vi "Blood Flow Measurement.vi"() -> ()   [LabVIEW 2023]
doc: "This example shows the application of the Time Frequency Analysis VIs in blood flow measurement. \n\nBlood velocity within a vessel is not uniform. Blood flow often has the maximum velocity at the center of a vessel and a zero velocity at the vascular wall. Blood velocity also changes over time. The complexity of the velocity distribution in a vessel is often associated with some arterial diseases. For example, when there is a high-grade stenosis within a femoral artery, the blood flow at the outlet of the stenosis usually has a velocity of a large mean, while the vortex or turbulence at the downstream generates a complicated velocity distribution. \n\nThe Doppler ultrasound technique has been widely applied to non-invasive blood flow measurement. The Doppler signals are generated by the backscattering from moving blood cells. The mean instantaneous frequency of the detected Doppler signal is proportional to the mean blood flow velocity in a vessel. The mean instantaneous bandwidth of the Doppler signal describes the velocity variation of the blood flow. \n\nThis example computes the time-frequency representation of a simulated Doppler signal and estimates the velocity and frequency bandwidth of the signal using the mean instantaneous frequency and mean instantaneous bandwidth of the time-frequency representation. This example uses the TFA STFT Spectrogram VI, the TFA Mean Instantaneous Frequency VI, and the TFA Mean Instantaneous Bandwidth VI.\n\n<b>Instruction:</b>\n1) Run this VI.\n2) Observe the measured mean velocity of blood flow. \n3) Browse the Block Diagram of this example to learn how to use TFA VIs in blood flow measurement."
uses:
  <vilib>/addons/Time Frequency Analysis/typedefs.llb/TFA Data.ctl
  <vilib>/addons/Time Frequency Analysis/Spectrogram.llb/TFA Fast Gabor Spectrogram (Complex).vi
  <vilib>/addons/Time Frequency Analysis/_control.llb/TFA Configure Spectrogram Indicator (Predefined Color Table).vi
  <vilib>/addons/_Advanced Signal Processing/NI_AdvSigProcTFA.lvlib
panel:
  out "aspt-left-top":bool
  out "Spectrogram":dbl[][](graph)
  out "Mean blood velocity and frequency bandwidth":cluster{"t0":dbl, "dt":dbl, "bandwidth":dbl[]}[](graph)
  out "Doppler Signal":dbl[][](graph)
  # "Overview: Shows the application of the Time Frequency Analysis VIs in blood flow measurement.\nRequirements: LabVIEW Full Development System, Advanced Signal Processing Toolkit\nInstructions: \n1. Run this VI.\n2. Observe the measured mean velocity of blood flow.  \n3. Browse the block diagram of this example to learn how to use Time Frequency Analysis VIs in blood flow measurement."
  # "Time Domain Signal"
  # "Time-Frequency Domain"
  # "Feature Extraction"
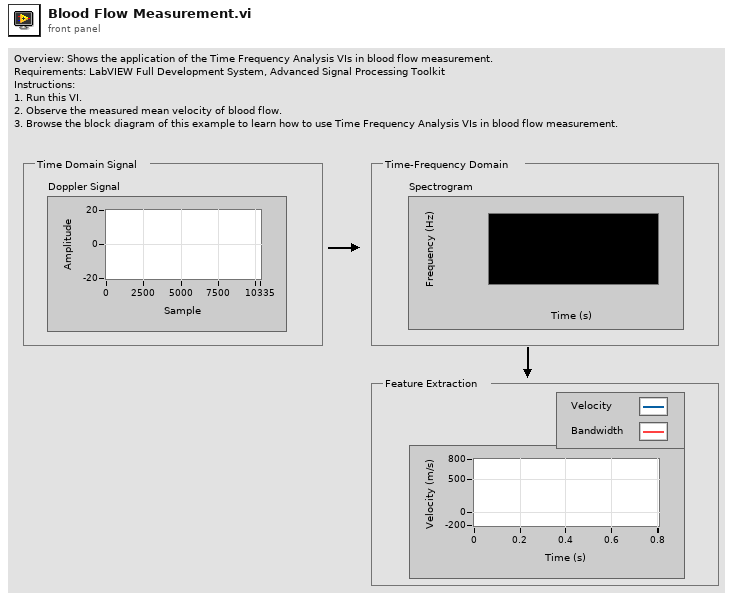
[diagram p1: front panel]
types:
  T1 = typedef "NI_AdvSigProcTFA.lvlib/TFA Data.ctl" = u16
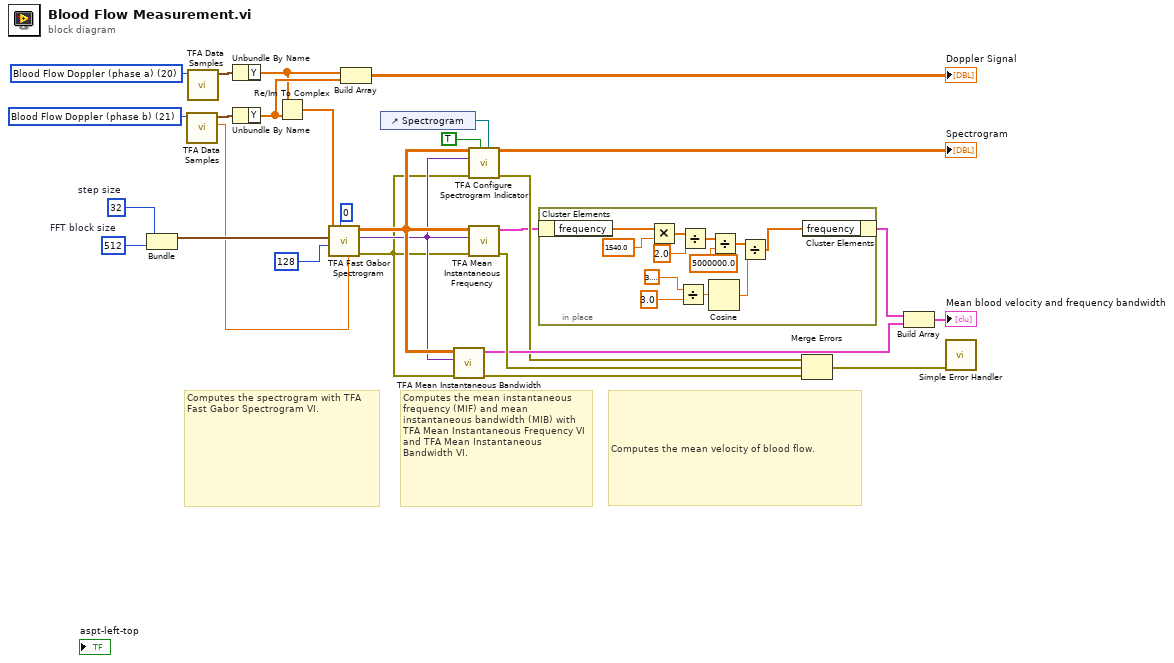
[diagram p0: block diagram]
diagram:
  w5 = T1 21 items=["PC Fan"=0, "Noisy Chirps"=1, "TDR 1"=2, "TDR 2"=3, "Liquefaction"=4, "Liquefaction Free"=5, "Aneurysm"=6, "Bat"=7, "RF"=8, "Two Gaussian"=9, "Three Gaussian"=10, "Chirp"=11, "Gaussian Chirp"=12, "Cross Chirp"=13, "Doppler"=14, "HOP"=15, "TF Sine"=16, "Three Tone"=17, "Four Tone"=23, "Blood Flow Doppler (phase a)"=20, "Blood Flow Doppler (phase b)"=21, "Heart sound"=22, "-"=18, "Random Noise"=19] ("data 2")
  w6 = T1 20 items=["PC Fan"=0, "Noisy Chirps"=1, "TDR 1"=2, "TDR 2"=3, "Liquefaction"=4, "Liquefaction Free"=5, "Aneurysm"=6, "Bat"=7, "RF"=8, "Two Gaussian"=9, "Three Gaussian"=10, "Chirp"=11, "Gaussian Chirp"=12, "Cross Chirp"=13, "Doppler"=14, "HOP"=15, "TF Sine"=16, "Three Tone"=17, "Four Tone"=23, "Blood Flow Doppler (phase a)"=20, "Blood Flow Doppler (phase b)"=21, "Heart sound"=22, "-"=18, "Random Noise"=19] ("data")
  w22 = 512  # FFT block size
  w21 = 32  # step size
  # "Computes the mean velocity of blood flow."
  # "Computes the mean instantaneous frequency (MIF) and mean instantaneous bandwidth (MIB) with TFA Mean Instantaneous Frequency VI and TFA Mean Instantaneous Bandwidth VI."
  # "Computes the spectrogram with TFA Fast Gabor Spectrogram VI."
  n1 = Bundle("step size"=w21, "FFT block size"=w22) -> (w20:cluster{"step size":i32, "FFT block size":i32})  [unwired: 1 out]
  n2 = call <vilib>:"TFA Data Samples.vi"("data"=w5) -> ("sampling rate"=w9:dbl, "signal"=w13:waveform(dbl))  [unwired: 9 out]
  n3 = call <vilib>:"TFA Data Samples.vi"("data"=w6) -> ("signal"=w14:waveform(dbl))  [unwired: 10 out]
  n4 = Unbundle By Name(w14) -> ("Y"=w10:dbl[])
  n5 = Unbundle By Name(w13) -> ("Y"=w11:dbl[])
  n6 = Re/Im To Complex(1:w11, 2:w10) -> (0:w12:cdb[])
  n7 = call-poly <vilib>:"TFA Fast Gabor Spectrogram.vi"("sampling rate"=w9, "order"=0, "Gaussian window length"=128, "time-frequency sampling info"=w20, "signal"=w12) -> ("error out"=w4:errorcluster, "scale info"=w18:variant, "spectrogram"=w19:dbl[][])  [unwired: 1 in, 3 out]
  n8 = Build Array(w10, w11) -> (→"Doppler Signal":dbl[][])
  n9 = control-ref of="Spectrogram"() -> (w16:refnum<vi>)
  n10 = call <vilib>:"TFA Mean Instantaneous Bandwidth.vi"("error in (no error)"=w4, "scale info"=w18, "spectrogram"=w19) -> ("error out"=w24:errorcluster, "MIB"=w26:cluster{"t0":dbl, "dt":dbl, "bandwidth":dbl[]})  [unwired: 7 out]
  n11 = call-poly <vilib>:"TFA Configure Spectrogram Indicator.vi"("reference of TF spectrogram indicator"=w16, "dB on? (F)"=TRUE ("dB? (F)"), "error in (no error)"=w4, "scale info"=w18, "spectrogram"=w19) -> ("error out"=w3:errorcluster, "TF spectrogram indicator"=→"Spectrogram":dbl[][])  [unwired: 2 in, 3 out]
  n12 = call <vilib>:"TFA Mean Instantaneous Frequency.vi"("error in (no error)"=w4, "scale info"=w18, "spectrogram"=w19) -> ("error out"=w28:errorcluster, "MIF"=w2:cluster{"t0":dbl, "dt":dbl, "frequency":dbl[]})  [unwired: 7 out]
  n13 = in-place {
    n14 = in-place-cluster #1(w2) -> ("frequency"=w30:dbl[])
    n15 = Multiply(x=w30, y=1540.0) -> (x*y=w39:dbl[])
    n16 = Divide(x=3.141592653589793 ("Pi"), y=3.0) -> (x/y=w31:dbl)
    n17 = Divide(x=w39, y=2.0) -> (x/y=w37:dbl[])
    n18 = Cosine(x=w31) -> (cos(x)=w34:dbl)
    n19 = Divide(x=w37, y=5000000.0 ("f0")) -> (x/y=w35:dbl[])
    n20 = Divide(x=w35, y=w34) -> (x/y=w29:dbl[])
    n21 = in-place-cluster #1("frequency"=w29) -> (w1:cluster{"t0":dbl, "dt":dbl, "frequency":dbl[]})
  }
  n22 = Merge Errors(w3, w28, w24) -> (w23:errorcluster)
  n23 = Build Array(w1, w26) -> (→"Mean blood velocity and frequency bandwidth":cluster{"t0":dbl, "dt":dbl, "bandwidth":dbl[]}[])
  n24 = call <vilib>:"Simple Error Handler.vi"("error in (no error)"=w23) -> ()  [unwired: 1 in, 8 out]
